vi "is_valid_ref.vi"(7 "raise error if invalid? (False)":bool, 8 "error in (no error)":errorcluster, 11 "Item in":refnum<class "Item.lvclass">) -> (0 "error out":errorcluster, 2 "ref_is_valid?":bool, 3 "Item out":refnum<class "Item.lvclass">)   [LabVIEW 2020, in "toml_edit.lvlib" / "Item.lvclass"]
uses:
  Item.lvclass
  Item.lvclass/Item.ctl
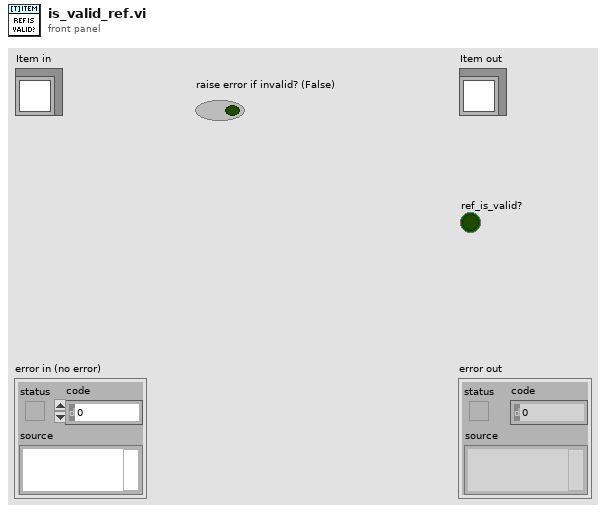
[diagram p1: front panel]
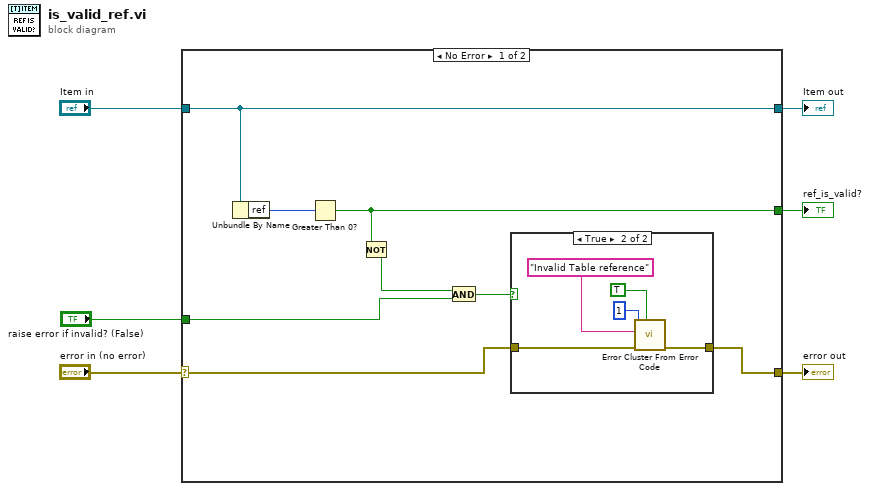
[diagram p0: block diagram]
diagram:
  n1 = case shown="No Error" "error in (no error)" {
    selector: "error in (no error)" -> [w10 w22]
    tunnel: [w9 w22] -> w5
    tunnel: [w14 w21] -> w3
    tunnel: "Item in" -> [w14 w21]
    tunnel: [w7 _] -> w2
    tunnel: "raise error if invalid? (False)" -> [w8 _]
    frame No Error {
      n2 = Unbundle By Name(w14) -> ("ref"=w13:u64)
      n3 = Greater Than 0?(x=w13) -> (x > 0?=w7:bool)
      n4 = Not(x=w7) -> (.not. x?=w11:bool)
      n5 = And(x=w11, y=w8) -> (x .and. y?=w12:bool)
      n6 = case shown="True" w12 {
        tunnel: [w15 w17] -> w9
        tunnel: w10 -> [w15 w16]
        frame False {
        }
        frame True {
          n7 = call <vilib>:"Error Cluster From Error Code.vi"("show call chain? (False)"=TRUE, "error in (no error)"=w16, "error message (\"\")"="Invalid Table reference" ("error message (\"\")"), "error code (0)"=1) -> ("error out"=w17:errorcluster)  [unwired: 5 in]
        }
      }
    }
    frame Error {
    }
  }
  "error out" <- w5
  "Item out" <- w3
  "ref_is_valid?" <- w2
